vi "Graph.UpdateAOs.vi"(8 "error in (no error)":errorcluster, 11 "AO Data [ ]":cluster{"AO Name":string, "AO Value":variant}[](array[cluster])) -> (0 "error out":errorcluster, 3 "Graph Data":cluster{"[0]":dbl, "[1]":dbl})   [LabVIEW 2013]
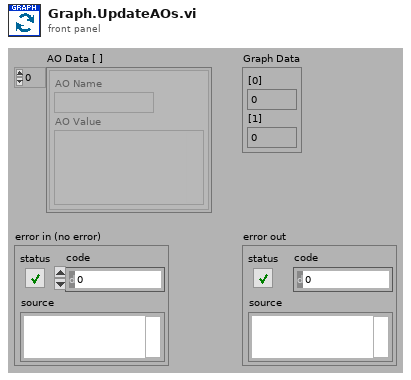
[diagram p1: front panel]
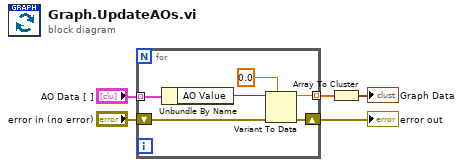
[diagram p0: block diagram]
diagram:
  n1 = for {
    tunnel: "AO Data [ ]" -> [w11] mode=indexing
    tunnel: [w8] -> w2 mode=indexing
    shift-right: [w6] -> w5
    shift-left: "error in (no error)" -> [w7]
    n2 = Unbundle By Name(w11) -> ("AO Value"=w10:variant)
    n3 = Variant To Data(error in=w7, type=0.0, Variant=w10) -> (data=w8:dbl, error out=w6:errorcluster)
  }
  "error out" <- w5
  n4 = Array To Cluster(array=w2) -> (cluster=→"Graph Data":cluster{"[0]":dbl, "[1]":dbl})
